vi "mxwScript_API_Option_SetConPanePattern.vi"(8 "error in (no error)":errorcluster, 9 "rotation":string, 10 "pattern":u32=4815, 11 "options in":T1[](array[typedef])) -> (0 "error out":errorcluster, 3 "options out":T1[](array[typedef]))   [LabVIEW 2017]
uses:
  codeGenAPISupport.llb/cgAPI_mxwScript_OptionData.ctl
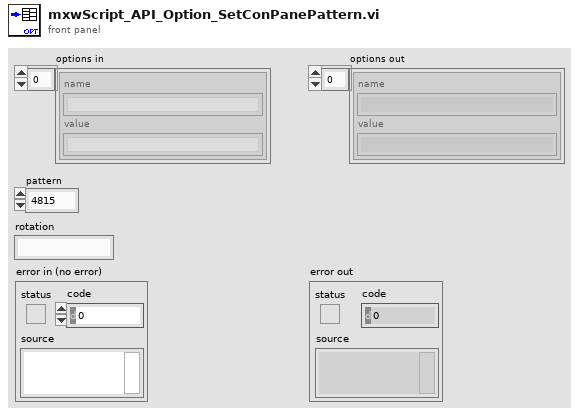
[diagram p1: front panel]
types:
  T1 = typedef "cgAPI_mxwScript_OptionData.ctl" = cluster{"name":string, "value":string}
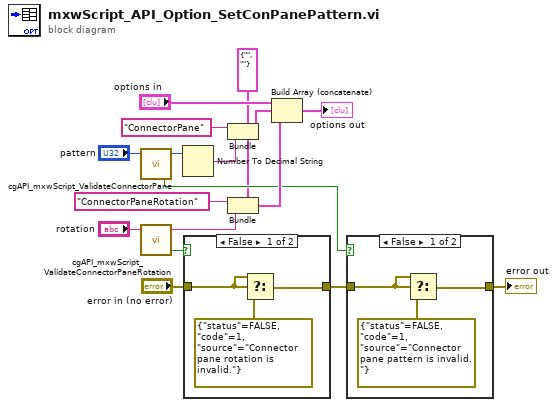
[diagram p0: block diagram]
diagram:
  w1 = T1 {"name"="", "value"=""} ("optionData")
  n1 = call "cgAPI_mxwScript_ValidateConnectorPane.vi"("pane"="pattern") -> ("valid?"=w2:bool, "validated pane"=w13:u32)  [unwired: 1 in, 2 out]
  n2 = call "cgAPI_mxwScript_ValidateConnectorPaneRotation.vi"("rotation"="rotation") -> ("valid?"=w6:bool, "validated rotation"=w9:string)  [unwired: 1 in, 2 out]
  n3 = Number To Decimal String(number=w13) -> (decimal integer string=w11:string)  [unwired: 1 out]
  n4 = case shown="False" w6 {
    tunnel: "error in (no error)" -> [w19 w21]
    tunnel: [w18 w21] -> w3
    frame False {
      n5 = Select(t=w19, s=w19, f=errorcluster {"status"=FALSE, "code"=1, "source"="Connector pane rotation is invalid."} ("error out 2")) -> (s? t:f=w18:errorcluster)
    }
    frame True {
    }
  }
  n6 = Bundle(cluster=w1, "name"="ConnectorPane" ("element"), "value"=w11) -> (w8:T1)
  n7 = Bundle(cluster=w1, "name"="ConnectorPaneRotation" ("element"), "value"=w9) -> (w7:T1)
  n8 = Build Array (concatenate)("options in", w8, w7) -> (→"options out":T1[])
  n9 = case shown="False" w2 {
    tunnel: w3 -> [w22 w25]
    tunnel: [w24 w25] -> w4
    frame False {
      n10 = Select(t=w22, s=w22, f=errorcluster {"status"=FALSE, "code"=1, "source"="Connector pane pattern is invalid."} ("error out 2")) -> (s? t:f=w24:errorcluster)
    }
    frame True {
    }
  }
  "error out" <- w4
